vi "Router - Close.vi"(8 "error in (no error)":errorcluster, 11 "Router Data":T1) -> (0 "error out":errorcluster)   [LabVIEW 2016, in "PXImc Router.lvlib"]
uses:
  PXImc Router.lvlib
  Controls/Router Data.ctl
  Controls/Reader Data.ctl
  Controls/Table Index-Size.ctl
  Controls/Writer Data.ctl
  <vilib>/pximc/nipximc.lvlib
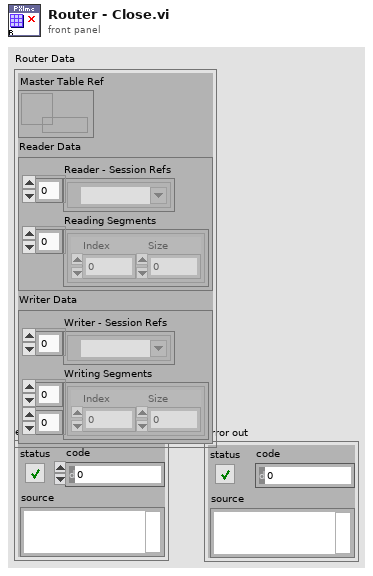
[diagram p1: front panel]
types:
  T1 = typedef "PXImc Router.lvlib/Router Data.ctl" = cluster{"Master Table Ref":refnum<data-value>, "Reader Data":T2, "Writer Data":T4}
  T2 = typedef "PXImc Router.lvlib/Reader Data.ctl" = cluster{"Reader - Session Refs":refnum<k21>[], "Reading Segments":T3[]}
  T3 = typedef "PXImc Router.lvlib/Table Index-Size.ctl" = cluster{"Index":u32, "Size":u32}
  T4 = typedef "PXImc Router.lvlib/Writer Data.ctl" = cluster{"Writer - Session Refs":refnum<k21>[], "Writing Segments":T3[][]}
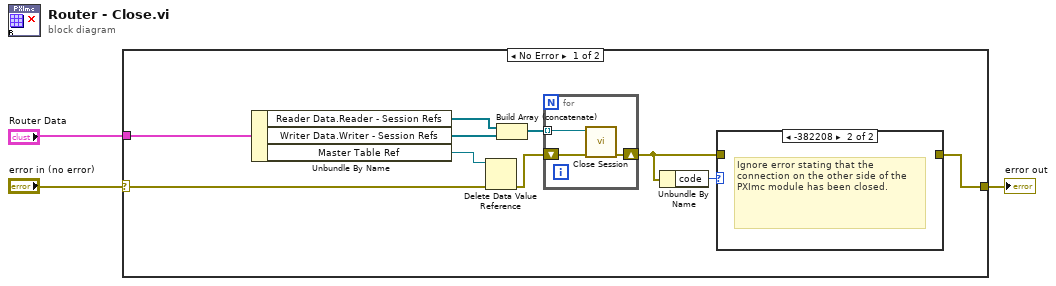
[diagram p0: block diagram]
diagram:
  n1 = case shown="No Error" "error in (no error)" {
    selector: "error in (no error)" -> [w5 w18]
    tunnel: [w9 w18] -> w3
    tunnel: "Router Data" -> [w4 _]
    frame No Error {
      n2 = Unbundle By Name(w4) -> ("Reader Data.Reader - Session Refs"=w8:refnum<k21>[], "Writer Data.Writer - Session Refs"=w7:refnum<k21>[], "Master Table Ref"=w6:refnum<data-value>)
      n3 = Delete Data Value Reference(data value reference=w6, error in=w5) -> (error out=w13:errorcluster)  [unwired: 1 out]
      n4 = Build Array (concatenate)(w8, w7) -> (w11:refnum<k21>[])
      n5 = for {
        tunnel: w11 -> [w16] mode=indexing
        shift-right: [w14] -> w12
        shift-left: w13 -> [w15]
        n6 = call <vilib>:"Close Session.vi"("error in (no error)"=w15, "session in"=w16) -> ("error out"=w14:errorcluster)  [unwired: 9 in]
      }
      n7 = Unbundle By Name(w12) -> ("code"=w10:i32)
      n8 = case shown="-382208" w10 {
        tunnel: w12 -> [w17 _]
        tunnel: [w17 _] -> w9
        frame 0, Default {
        }
        frame -382208 {
          # "Ignore error stating that the connection on the other side of the PXImc module has been closed."
        }
      }
    }
    frame Error {
    }
  }
  "error out" <- w3
